vi "MsgBox - Get Messages from Excel.vi"() -> ()   [LabVIEW 2013]
uses:
  <vilib>/Utility/NIReport.llb/NI_report.lvclass
  <vilib>/addons/_office/excel.llb/Excel Get Data ([str]).vi
  <vilib>/addons/_office/NI_ReportGenerationToolkit.lvlib
  <vilib>/Utility/NIReport.llb/Excel/NI_Excel.lvclass
panel:
  in  "data type":string[][](array[string])
  out "Config.Messages":string[][](array[string])
  in  "template (empty)":path
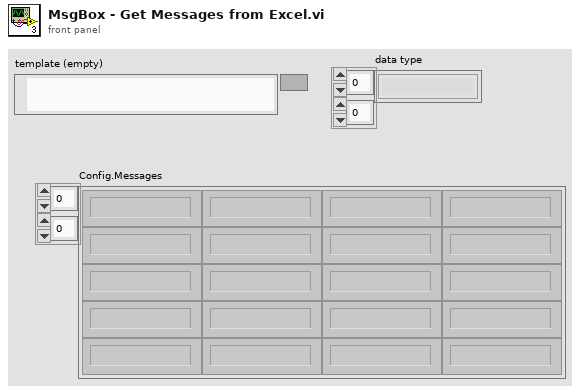
[diagram p1: front panel]
types:
  T1 = enum16{"maximized", "minimized", "normal", "no change"}
  T2 = enum16{"Standard Report", "HTML", "Word", "Excel"}
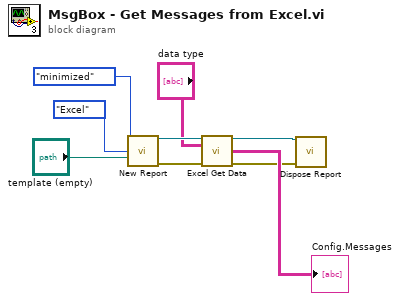
[diagram p0: block diagram]
diagram:
  n1 = call <vilib>:"New Report.vi"("window state (normal)"=T1."minimized", "report type"=T2."Excel", "template (empty)"="template (empty)") -> ("report out"=w9:refnum<class "NI_report.lvclass">, "error out"=w8:errorcluster)  [unwired: 11 in]
  n2 = call-poly <vilib>:"Excel Get Data.vi"("report in"=w9, "data type"="data type", "error in (no error)"=w8) -> ("report out"=w4:refnum<class "NI_report.lvclass">, "data"=→"Config.Messages":string[][], "error out"=w5:errorcluster)  [unwired: 10 in]
  n3 = call-dynamic "Dispose Report.vi"("report in"=w4, "error in (no error)"=w5) -> ()  [unwired: 13 in, 1 out]
